vi "Cal Inst current voltage waveforms.vi"(8 "error in (no error)":errorcluster, 11 "VISA resource name":refnum<visa-resource-name>) -> (0 "error out":errorcluster, 2 "Waveform Graph":waveform(sgl)[](graph), 3 "VISA resource name out":refnum<visa-resource-name>)   [LabVIEW 2013]
uses:
  Libraries/California Instruments iX Series/California Instruments iX Series.lvlib
panel:
  out "read buffer":string
  out "Waveform Graph 3":sgl[](graph)
  out "return count 3":u32
  out "Number of Bytes at Port":u32
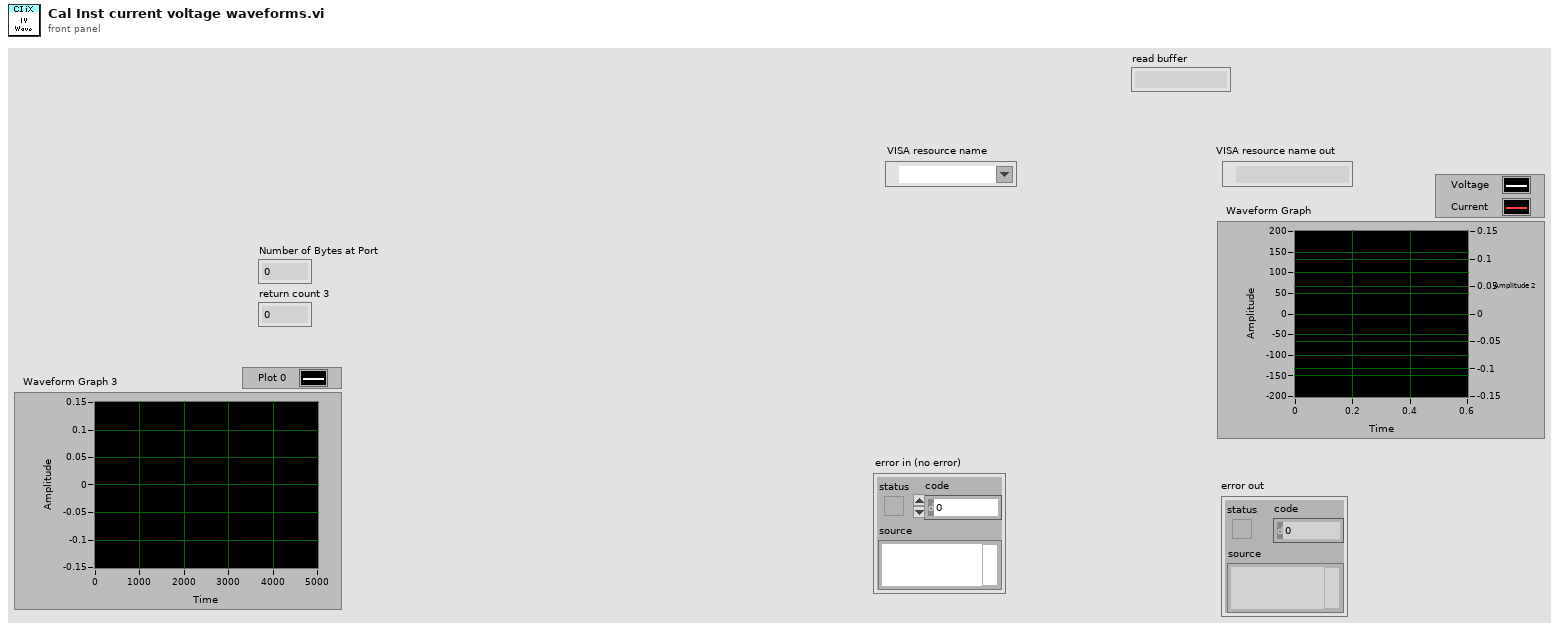
[diagram p1: front panel]
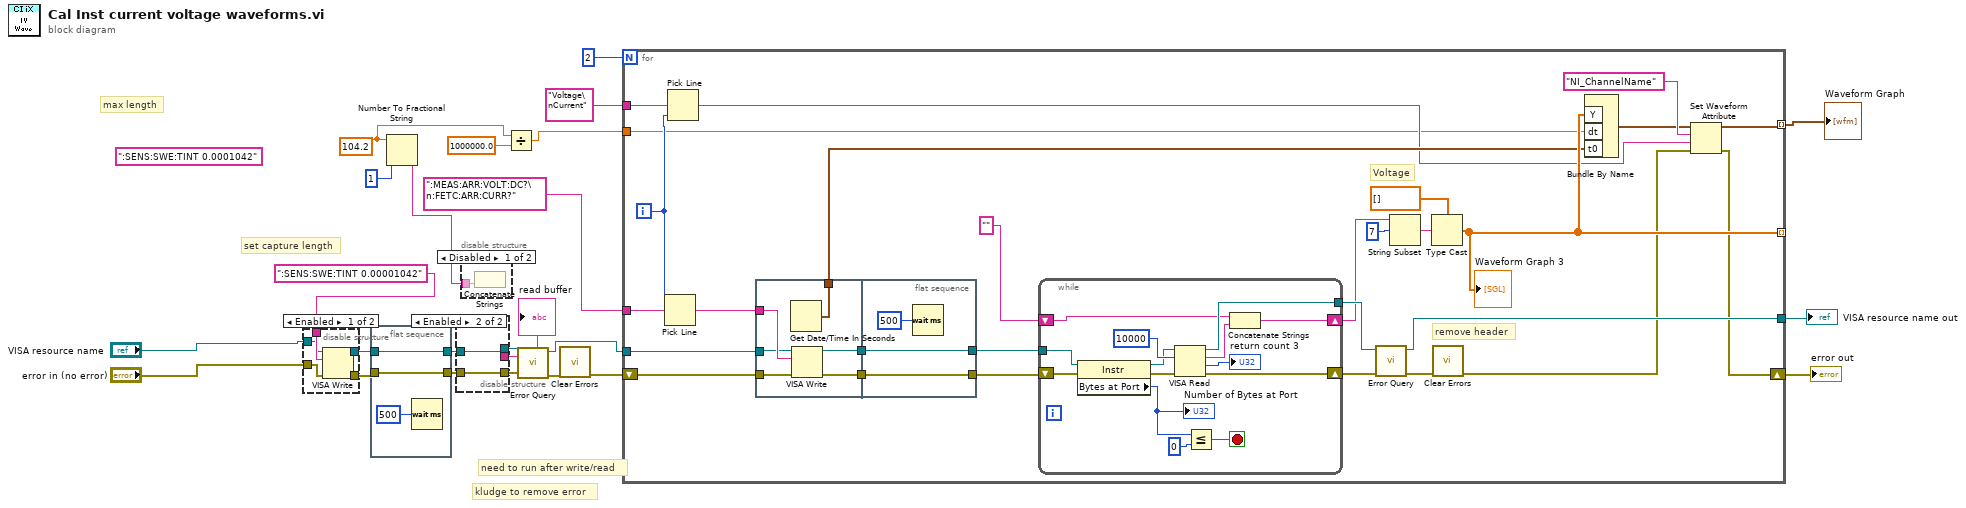
[diagram p0: block diagram]
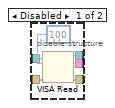
[diagram p3: hidden frame]
diagram:
  (unwired) ":SENS:SWE:TINT 0.0001042" ("multi-line string")
  w16 = 104.2
  # "max length"
  # "kludge to remove error"
  # "need to run after write/read"
  # "set capture length"
  n1 = disable-structure shown="Enabled" {
    disable-tunnel: [w29 w30] -> w10
    disable-tunnel: [w28 w31] -> w9
    disable-tunnel: ":SENS:SWE:TINT 0.00001042" ("multi-line string") -> [w27 _]
    disable-tunnel: "VISA resource name" -> [w26 w31]
    disable-tunnel: "error in (no error)" -> [w25 w30]
    frame Enabled {
      n2 = VISA Write(VISA resource name=w26, write buffer=w27, error in (no error)=w25) -> (VISA resource name out=w28:refnum<visa-resource-name>, error out=w29:errorcluster)  [unwired: 1 out]
    }
    frame Disabled {
    }
  }
  n3 = flat-sequence {
    tunnel: w10 -> [w33]
    tunnel: [w33] -> w8
    tunnel: w9 -> [w32]
    tunnel: [w32] -> w7
    frame #0 {
      n4 = Wait (ms)(milliseconds to wait=u32 500) -> ()  [unwired: 1 out]
    }
  }
  n5 = Number To Fractional String(number=w16, precision (6)=i16 1) -> (F-format string=w18:string)  [unwired: 2 in]
  n6 = disable-structure shown="Enabled" {
    disable-tunnel: w8 -> [w40 w41]
    disable-tunnel: w7 -> [w39 w42]
    disable-tunnel: [w38 w42] -> w6
    disable-tunnel: [w37 w41] -> w5
    disable-tunnel: [w36 _] -> w4
    frame Disabled {
      n7 = VISA Read(VISA resource name=w39, byte count=u32 100, error in (no error)=w40) -> (VISA resource name out=w38:refnum<visa-resource-name>, read buffer=w36:string, error out=w37:errorcluster)  [unwired: 1 out]
    }
    frame Enabled {
    }
  }
  "read buffer" <- w4
  n8 = disable-structure shown="Disabled" {
    disable-tunnel: w18 -> [w43 _]
    frame Disabled {
      n9 = Concatenate Strings(w43) -> ()  [unwired: 1 in, 1 out]
    }
    frame Enabled {
    }
  }
  n10 = Divide(x=w16, y=1000000.0) -> (x/y=w15:dbl)
  n11 = call "Error Query.vi"("error in (no error)"=w5, "VISA resource name"=w6) -> ("error out"=w13:errorcluster, "VISA resource name out"=w12:refnum<visa-resource-name>)  [unwired: 6 in, 2 out]
  n12 = call <vilib>:"Clear Errors.vi"("error in (no error)"=w13) -> ("error out"=w11:errorcluster)  [unwired: 6 in]
  n13 = for {
    N: 2 -> [_]
    tunnel: ":MEAS:ARR:VOLT:DC?\n:FETC:ARR:CURR?" ("multi-line string") -> [w67]
    tunnel: [w59] -> _ mode=indexing
    shift-right: [w45] -> w22
    shift-left: w11 -> [w53]
    tunnel: [w62] -> w21
    tunnel: w12 -> [w57]
    tunnel: "Voltage\nCurrent" ("multi-line string") -> [w50]
    tunnel: [w47] -> w19 mode=indexing
    tunnel: w15 -> [w44]
    i -> [w49]
    # "Voltage"
    # "remove header"
    n14 = Pick Line(multi-line string=w67, line index=w49) -> (output string=w58:string)  [unwired: 1 in]
    n15 = Pick Line(multi-line string=w50, line index=w49) -> (output string=w48:string)  [unwired: 1 in]
    n16 = flat-sequence {
      tunnel: w58 -> [w91]
      tunnel: w57 -> [w90]
      tunnel: [w89] -> w56
      tunnel: [w88] -> w54
      tunnel: w53 -> [w87]
      tunnel: [w86] -> w52
      tunnel: w56 -> [w93]
      tunnel: [w93] -> w55
      tunnel: [w92] -> w51
      tunnel: w52 -> [w92]
      frame #0 {
        n17 = Get Date/Time In Seconds() -> (seconds since 1Jan1904=w88:timestamp)
        n18 = VISA Write(VISA resource name=w90, write buffer=w91, error in (no error)=w87) -> (VISA resource name out=w89:refnum<visa-resource-name>, error out=w86:errorcluster)  [unwired: 1 out]
      }
      frame #1 {
        n19 = Wait (ms)(milliseconds to wait=u32 500) -> ()  [unwired: 1 out]
      }
    }
    n20 = while {
      tunnel: [w84] -> w69
      shift-right: [w73] -> w63
      shift-left: "" -> [w82]
      shift-right: [w77] -> w70
      shift-left: w51 -> [w78]
      tunnel: w55 -> [w72]
      stop <- w74 stop-if-true
      n21 = property class="Instr"(reference=w72, error in=w78) -> (reference out=w80:refnum<visa-resource-name>, error out=w79:errorcluster, "Bytes at Port"=w76:u32)
      "Number of Bytes at Port" <- w76
      n22 = VISA Read(VISA resource name=w80, byte count=u32 10000, error in (no error)=w79) -> (VISA resource name out=w84:refnum<visa-resource-name>, read buffer=w81:string, return count=→"return count 3":u32, error out=w77:errorcluster)
      n23 = Less Or Equal?(x=w76, y=u32 0) -> (x <= y?=w74:bool)
      n24 = Concatenate Strings(w82, w81) -> (w73:string)
    }
    n25 = call "Error Query.vi"("error in (no error)"=w70, "VISA resource name"=w69) -> ("error out"=w71:errorcluster, "VISA resource name out"=w62:refnum<visa-resource-name>)  [unwired: 6 in, 2 out]
    n26 = String Subset(string=w63, offset (0)=7) -> (substring=w65:string)  [unwired: 1 in]
    n27 = Type Cast(type=sgl[] [], x=w65) -> (*(type *) &x=w59:sgl[])
    "Waveform Graph 3" <- w59
    n28 = call <vilib>:"Clear Errors.vi"("error in (no error)"=w71) -> ("error out"=w46:errorcluster)  [unwired: 6 in]
    n29 = Bundle By Name("Y"=w59, "dt"=w44, "t0"=w54) -> (w60:waveform(sgl))  [unwired: 1 in]
    n30 = Set Waveform Attribute(4:w46, 5:w48, 6:"NI_ChannelName" ("name"), 7:w60) -> (0:w45:errorcluster, 3:w47:waveform(sgl))  [unwired: 1 out]
  }
  "Waveform Graph" <- w19
  "error out" <- w22
  "VISA resource name out" <- w21
